vi "TestiLabview2.vi"() -> ()   [LabVIEW 2018]
panel:
  out "Isbjerg spottet":i32[](array[numeric])
  out "Y":dbl[][](array[numeric])
  out "X":dbl[][](array[numeric])
  out "Image":T1(plugin-control)
  out "Array":cluster{"X Centroid":sgl, "Y Centroid":sgl}[](array[cluster])
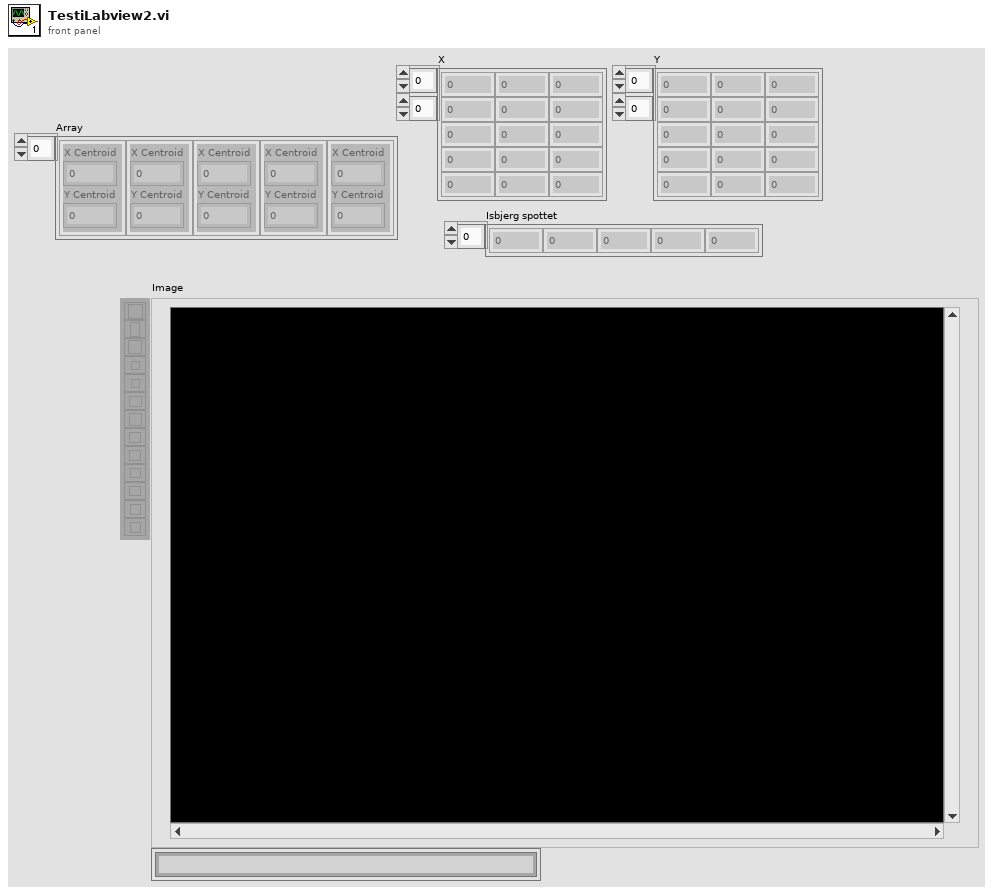
[diagram p1: front panel]
types:
  T1 = typedef "IMAQ Image.ctl" = refnum<image>
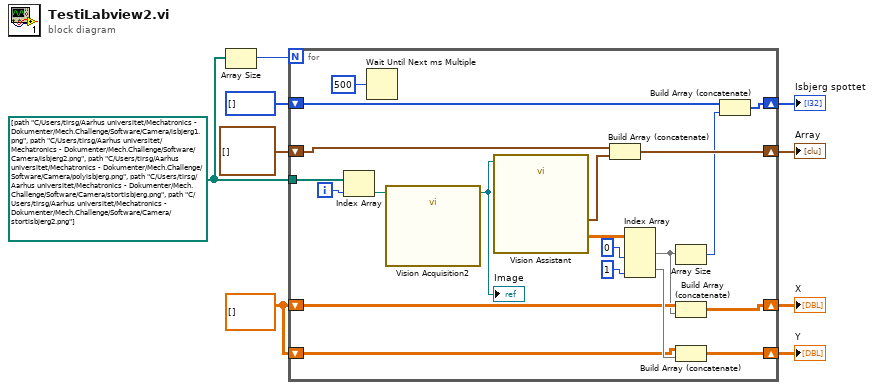
[diagram p0: block diagram]
diagram:
  w7 = dbl[][] []
  w3 = path[] [path "C:/Users/tirsg/Aarhus universitet/Mechatronics - Dokumenter/Mech.Challenge/Software/Camera/isbjerg1.png", path "C:/Users/tirsg/Aarhus universitet/Mechatronics - Dokumenter/Mech.Challenge/Software/Camera/isbjerg2.png", path "C:/Users/tirsg/Aarhus universitet/Mechatronics - Dokumenter/Mech.Challenge/Software/Camera/polyisbjerg.png", path "C:/Users/tirsg/Aarhus universitet/Mechatronics - Dokumenter/Mech.Challenge/Software/Camera/stortisbjerg.png", path "C:/Users/tirsg/Aarhus universitet/Mechatronics - Dokumenter/Mech.Challenge/Software/Camera/stortisbjerg2.png"] ("appended array")
  n1 = Array Size(array=w3) -> (size(s)=w2:i32)
  n2 = for {
    N: w2 -> [_]
    shift-right: [w29] -> w9
    shift-left: cluster{"X Centroid":sgl, "Y Centroid":sgl}[] [] -> [w27]
    tunnel: w3 -> [w25]
    shift-right: [w18] -> w6
    shift-left: w7 -> [w16]
    shift-right: [w17] -> w5
    shift-left: w7 -> [w15]
    shift-right: [w12] -> w1
    shift-left: i32[] [] -> [w11]
    i -> [w26]
    n3 = Index Array(array=w25, index=w26) -> (element=w24:path)
    n4 = Wait Until Next ms Multiple(millisecond multiple=u32 500) -> ()  [unwired: 1 out]
    n5 = call "Vision Acquisition2"("Image Path"=w24) -> ("Image Out"=w10:T1)  [unwired: 25 in, 1 out]
    "Image" <- w10
    n6 = call "Vision Assistant"("Image In"=w10) -> ("Centroid (Centroid 1)"=w28:cluster{"X Centroid":sgl, "Y Centroid":sgl}, "Particle Measurements (Pixels) (Particle Analysis 1)"=w20:dbl[][])  [unwired: 23 in, 2 out]
    n7 = Build Array (concatenate)(w27, w28) -> (w29:cluster{"X Centroid":sgl, "Y Centroid":sgl}[])
    n8 = Index Array(array=w20, index (col) #1=0 ("index (col)"), index (col) #2=1 ("index (col)")) -> (element #1=w14:dbl[], element #2=w19:dbl[])  [unwired: 2 in]
    n9 = Array Size(array=w14) -> (size(s)=w13:i32)
    n10 = Build Array (concatenate)(w16, w14) -> (w18:dbl[][])
    n11 = Build Array (concatenate)(w15, w19) -> (w17:dbl[][])
    n12 = Build Array (concatenate)(w11, w13) -> (w12:i32[])
  }
  "Array" <- w9
  "X" <- w6
  "Y" <- w5
  "Isbjerg spottet" <- w1
